vi "Write Command ID.vi"(8 "error in (no error)":errorcluster, 10 "Command ID":u32, 11 "Command in":refnum<class "Command Actor.lvclass">) -> (0 "error out":errorcluster, 3 "Command out":refnum<class "Command Actor.lvclass">)   [LabVIEW 2014, in "Robot Actor Framework.lvlib" / "Command Actor.lvlib" / "Command Actor.lvclass"]
uses:
  Command Actor.lvclass
  Command Actor.lvclass/Command Actor.ctl
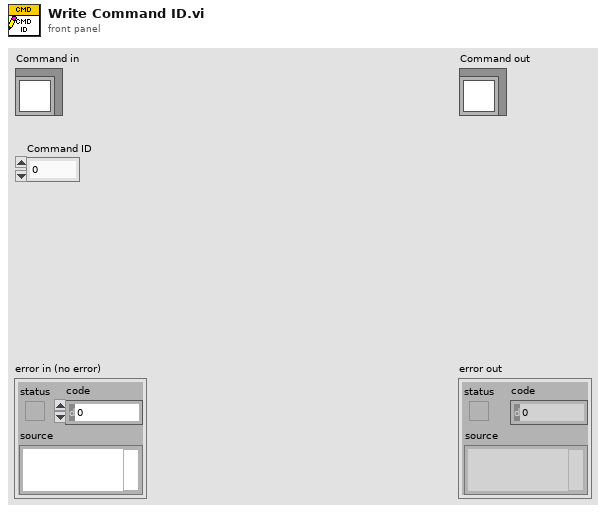
[diagram p1: front panel]
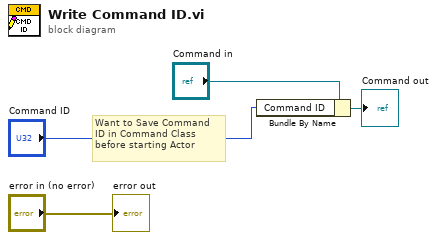
[diagram p0: block diagram]
diagram:
  # "Want to Save Command\nID in Command Class\nbefore starting Actor"
  n1 = Bundle By Name(cluster="Command in", "Command ID"="Command ID") -> (→"Command out":refnum<class "Command Actor.lvclass">)
  "error out" <- "error in (no error)"
